vi "ConvertProgramRegisterToString.vi"(11 "Program Register":T1) -> (3 "Register":string)   [LabVIEW 2012, in "Keithley-2602.lvlib"]
uses:
  Keithley-2602.lvlib
  Public/Controls/ProgramRegister.ctl
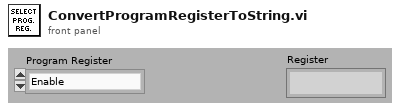
[diagram p1: front panel]
types:
  T1 = typedef "Keithley-2602.lvlib/ProgramRegister.ctl" = enum16{"Enable", "Positive Transition", "Negative Transition"}
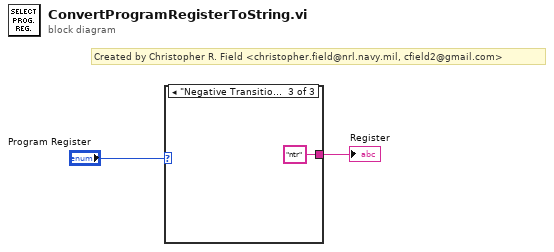
[diagram p0: block diagram]
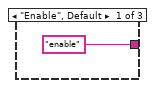
[diagram p2: hidden frame]
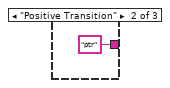
[diagram p3: hidden frame]
diagram:
  # "Created by Christopher R. Field <christopher.field@nrl.navy.mil, cfield2@gmail.com>"
  n1 = case shown="\"Negative Transition\"" "Program Register" {
    tunnel: ["enable" "ptr" "ntr"] -> w2
    frame "Enable", Default {
    }
    frame "Positive Transition" {
    }
    frame "Negative Transition" {
    }
  }
  "Register" <- w2
